vi "permissions_set.vi"   [LabVIEW 2015, in "lv-bin-windows.lvlib" / "v1.lvlib"]
uses:
  v1.lvlib
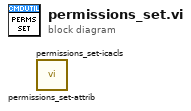
[diagram p0: block diagram]
diagram:
  n1 = call "permissions_set-attrib.vi"() -> ()  [unwired: 10 in, 2 out]
  n2 = call "permissions_set-icacls.vi"() -> ()  [unwired: 10 in, 2 out]
